vi "Get Drivers List.vi"(11 "error in":errorcluster) -> (4 "drivers list out":string[](array[string]), 6 "total driver list":i32, 8 "removed duplicates":string[](array[string]), 10 "removed duplicates size":i32, 14 "total size":i32, 15 "error out":errorcluster)   [LabVIEW 2021, in "Converter Reusables.lvlib"]
uses:
  Converter Reusables.lvlib
  TypeDefs/Dictionary States.ctl
  77a78234-7449-441e-9ac3-41e4d218bce4.vi
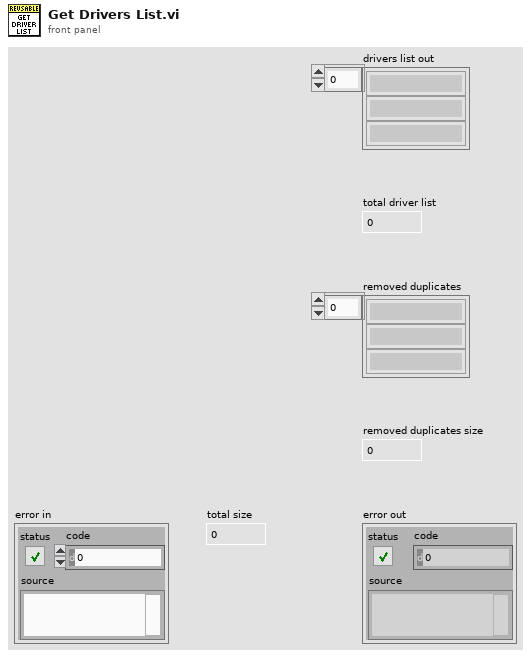
[diagram p1: front panel]
types:
  T1 = typedef "Converter Reusables.lvlib/Dictionary States.ctl" = enum16{"Set", "Get", "Delete", "Delete All"}
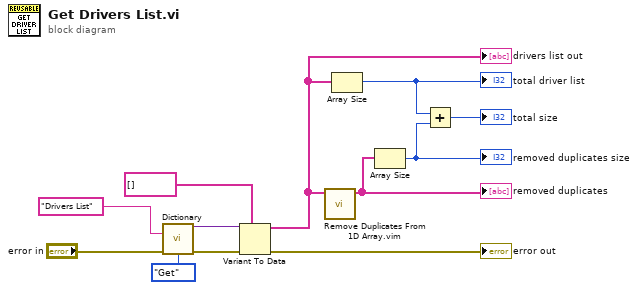
[diagram p0: block diagram]
diagram:
  n1 = call "Dictionary.vi"("key"="Drivers List" ("Key"), "error in"="error in", "dict states"=Dictionary_States."Get" ("Dict States")) -> ("variant out"=w8:variant, "error out"=w9:errorcluster)  [unwired: 11 in]
  n2 = Variant To Data(error in=w9, type=string[] [], Variant=w8) -> (data=w5:string[], error out=→"error out":errorcluster)
  "drivers list out" <- w5
  n3 = call "Remove Duplicates From 1D Array.vim"("array"=w5) -> ("array with duplicates removed"=w4:string[])  [unwired: 10 in]
  "removed duplicates" <- w4
  n4 = Array Size(array=w5) -> (size(s)=w3:i32)
  "total driver list" <- w3
  n5 = Array Size(array=w4) -> (size(s)=w2:i32)
  "removed duplicates size" <- w2
  n6 = Add(x=w3, y=w2) -> (x+y=→"total size":i32)
